vi "DelayGenerator.vi"(8 "error in (no error)":errorcluster, 11 "Time Stamp":timestamp) -> (0 "error out":errorcluster, 3 "DelayTarget":T1)   [LabVIEW 2009, in "DelayGenerator.lvlib"]
uses:
  DelayGenerator.lvlib
  Controls/DelayTarget.ctl
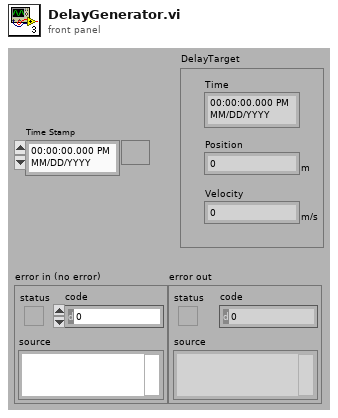
[diagram p1: front panel]
types:
  T1 = typedef "DelayTarget.ctl" = cluster{"Time":timestamp, "Position":dbl[unit], "Velocity":dbl[unit]}
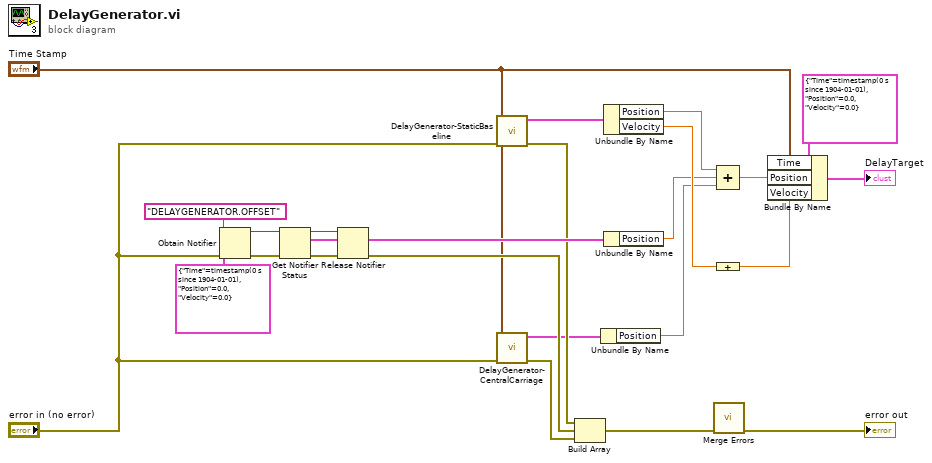
[diagram p0: block diagram]
diagram:
  n1 = Obtain Notifier(name (unnamed)="DELAYGENERATOR.OFFSET", notification data type=T1 {"Time"=timestamp(0 s since 1904-01-01), "Position"=0.0, "Velocity"=0.0} ("DelayTarget"), error in (no error)="error in (no error)") -> (notifier out=w17:refnum<notifier>, error out=w16:errorcluster)  [unwired: 1 in, 1 out]
  n2 = Get Notifier Status(notifier=w17, error in (no error)=w16) -> (notifier out=w15:refnum<notifier>, current notification=w13:T1, error out=w14:errorcluster)  [unwired: 2 out]
  n3 = Release Notifier(notifier=w15, error in (no error)=w14) -> (error out=w9:errorcluster)  [unwired: 1 in, 2 out]
  n4 = call "DelayGenerator-StaticBaseline.vi"("Time Stamp"="Time Stamp", "error in (no error)"="error in (no error)") -> ("DelayTarget"=w22:T1, "error out"=w10:errorcluster)  [unwired: 6 in]
  n5 = call "DelayGenerator-CentralCarriage.vi"("Time Stamp"="Time Stamp", "error in (no error)"="error in (no error)") -> ("DelayTarget"=w5:T1, "error out"=w6:errorcluster)  [unwired: 6 in]
  n6 = Build Array(w10, w9, w6) -> (w8:errorcluster[])
  n7 = Unbundle By Name(w5) -> ("Position"=w4:dbl[unit])
  n8 = Unbundle By Name(w22) -> ("Position"=w24:dbl[unit], "Velocity"=w23:dbl[unit])
  n9 = Unbundle By Name(w13) -> ("Position"=w12:dbl[unit])
  n10 = call <vilib>:"Merge Errors.vi"("error array in"=w8) -> ("error out"=→"error out":errorcluster)  [unwired: 6 in]
  n11 = Compound Arithmetic op=ADD(w24, w12, w4) -> (w21:dbl[unit])
  n12 = Compound Arithmetic op=ADD(w23) -> (w20:dbl[unit])
  n13 = Bundle By Name(cluster=T1 {"Time"=timestamp(0 s since 1904-01-01), "Position"=0.0, "Velocity"=0.0} ("DelayTarget"), "Time"="Time Stamp", "Position"=w21, "Velocity"=w20) -> (→"DelayTarget":T1)
